vi "Exercise 6.1 RT PID-DataLog - LED.vi"() -> ()   [LabVIEW 2014]
doc: "This example demonstrates how to simulate a general PID controller with alarms."
uses:
  <vilib>/platform/TimedLoop/XDataNode/XDataNode.xnode
  <vilib>/Platform/TimedLoop/XDataNode/nitl_modes.ctl
  <vilib>/Platform/TimedLoop/XDataNode/XDNodeRunTimeDep.lvlib
  <vilib>/Platform/TimedLoop/XDataNode/wakeup.ctl
  <vilib>/Platform/TimedLoop/XDataNode/timing_clust.ctl
  <vilib>/Utility/file.llb/Write To Spreadsheet File (DBL).vi
  <vilib>/NI/Current Value Table/Current Value Table.lvlib
  <vilib>/NI/Current Value Table/Type Defs/File Format.ctl
  <vilib>/NI/Current Value Table/DataTypes/Double_Read.vi
  <vilib>/NI/Current Value Table/DataTypes/Double_Write.vi
  <vilib>/NI/Current Value Table/DataTypes/Boolean_Write.vi
  <vilib>/NI/Current Value Table/DataTypes/Boolean_Read.vi
  <vilib>/NI/STM/NI STM.lvlib
  <vilib>/NI/STM/TCP/Write Message (TCP).vi
  <vilib>/Q-Wave Systems/QwaveSys RPi Training Package (Demo)/Exercises/Exercise 6 Network Communucation/LogData.vi
  <vilib>/Utility/file.llb/Write To Spreadsheet File (string).vi
  <vilib>/Q-Wave Systems/QwaveSys RPi Training Package (Demo)/Addons/QwaveSys RPi Training Library.lvlib
  <vilib>/NI/STM/TCP/Write Meta Data (TCP Ref).vi
  <vilib>/NI/STM/TCP/Get Connection Reference (TCP).vi
  <vilib>/NI/Current Value Table/Type Defs/Tag Grouping set.ctl
  <vilib>/NI/Current Value Table/Type Defs/Data Types.ctl
  <vilib>/NI/Current Value Table/Type Defs/Single Tag.ctl
  <vilib>/Q-Wave Systems/QwaveSys RPi Training Package (Demo)/Addons/WiringPi/WiringPi Pin Mode.ctl
  <vilib>/Q-Wave Systems/QwaveSys RPi Training Package (Demo)/Addons/WiringPi/WiringPi GPIO TypeDef.ctl
panel:
  in  "Data Log Rate (ms)":u32=5000
  out "DataLog Loop stop":bool
  out "Network Loop stop":bool
  out "PID Loop stop":bool
  out "Data Log Loop ms":u32=5001
  out "Network Loop ms":u32=100
  out "PID Loop ms":u32=20
  in  "stop":bool
  in  "LED2":T1=5 items=["Pin1_3.3V"=51, "Pin2_5V"=52, "Pin3_GPIO8_I2C1_SDA"=8, "Pin4_5V"=53, "Pin5_GPIO9_I2C1_SCL"=9, "Pin6_Gnd"=54, "Pin7_GPIO7_GPCLK0"=7, "Pin8_GPIO15_TXD_UART"=15, "Pin9_Gnd"=55, "Pin10_GPIO16_RXD_UART"=16, "Pin11_GPIO0"=0, "Pin12_GPIO1_PCMCLK_PWM0"=1, "Pin13_GPIO2"=2, "Pin14_Gnd"=56, "Pin15_GPIO3"=3, "Pin16_GPIO4"=4, "Pin17_3V"=57, "Pin18_GPIO5"=5, "Pin19_GPIO12_MOSI(SPI)"=12, "Pin20_Gnd"=58, "Pin21_GPIO13_MISO(SPI)"=13, "Pin22_GPIO6"=6, "Pin23_GPIO14_CLK(SPI)"=14, "Pin24_GPIO10_CE0_SPI"=10, "Pin25_Gnd"=59, "Pin26_GPIO11_CE1_SPI"=11, "Pin27_SDA0_I2C_EEPROM"=60, "Pin28_SCL0_I2C_EEPROM"=61, "Pin_29_GPIO21_GPCLK1"=21, "Pin30_Gnd"=62, "Pin31_GPIO22_GPCLK2"=22, "Pin32_GPIO26_PWM0"=26, "Pin33_GPIO23_PWM1"=23, "Pin34_Gnd"=63, "Pin35_GPIO24_PCMFS_PWM1"=24, "Pin36_GPIO27"=27, "Pin37_GPIO25"=25, "Pin38_GPIO28_PCM_DIN"=28, "Pin39_Gnd"=64, "Pin40_GPIO29_PCM_DOUT"=29]
  in  "LED1":T1=1 items=["Pin1_3.3V"=51, "Pin2_5V"=52, "Pin3_GPIO8_I2C1_SDA"=8, "Pin4_5V"=53, "Pin5_GPIO9_I2C1_SCL"=9, "Pin6_Gnd"=54, "Pin7_GPIO7_GPCLK0"=7, "Pin8_GPIO15_TXD_UART"=15, "Pin9_Gnd"=55, "Pin10_GPIO16_RXD_UART"=16, "Pin11_GPIO0"=0, "Pin12_GPIO1_PCMCLK_PWM0"=1, "Pin13_GPIO2"=2, "Pin14_Gnd"=56, "Pin15_GPIO3"=3, "Pin16_GPIO4"=4, "Pin17_3V"=57, "Pin18_GPIO5"=5, "Pin19_GPIO12_MOSI(SPI)"=12, "Pin20_Gnd"=58, "Pin21_GPIO13_MISO(SPI)"=13, "Pin22_GPIO6"=6, "Pin23_GPIO14_CLK(SPI)"=14, "Pin24_GPIO10_CE0_SPI"=10, "Pin25_Gnd"=59, "Pin26_GPIO11_CE1_SPI"=11, "Pin27_SDA0_I2C_EEPROM"=60, "Pin28_SCL0_I2C_EEPROM"=61, "Pin_29_GPIO21_GPCLK1"=21, "Pin30_Gnd"=62, "Pin31_GPIO22_GPCLK2"=22, "Pin32_GPIO26_PWM0"=26, "Pin33_GPIO23_PWM1"=23, "Pin34_Gnd"=63, "Pin35_GPIO24_PCMFS_PWM1"=24, "Pin36_GPIO27"=27, "Pin37_GPIO25"=25, "Pin38_GPIO28_PCM_DIN"=28, "Pin39_Gnd"=64, "Pin40_GPIO29_PCM_DOUT"=29]
  in  "Pin Mode":T2=enum."OUTPUT"
  in  "MIN":dbl(slide)=25.510204081632654 scale=0.0..100.0
  in  "MAX":dbl(slide)=74.48979591836735 scale=0.0..100.0
  out "Low Limit":bool
  out "High Limit":bool
  in  "SP:":dbl(slide)=54.966887417218544 min=0.0 max=0.0 scale=0.0..100.0
  out "MV:":dbl(slide)=100.0 scale=-100.0..100.0
  out "PV:":dbl(slide)=33.01408837398299 scale=0.0..100.0
  in  "PID gains":T3={"proportional gain (Kc)"=20.0, "integral time (Ti, min)"=0.008, "derivative time (Td, min)"=0.001} {"derivative time (Td, min)" format="%.3f"; "integral time (Ti, min)" format="%.3f"; "proportional gain (Kc)" format="%.3f"}
  # "Overview: This example demonstrates how to simulate a general PID controller with alarms.\nInstructions:\n1. Run the VI and observe the Process Variable (PV) following the Setpoint (SP) value.\n2. Move the setpoint above or below the High Limit (HL) or Low Limit (LL). Verify the controls flashing when limits are reached.\n3. Change the Alarm limits to a value above or below if you are changing HL or LL, respectively and verify that the controller stop flashing.\n3. Click Stop to stop the VI."
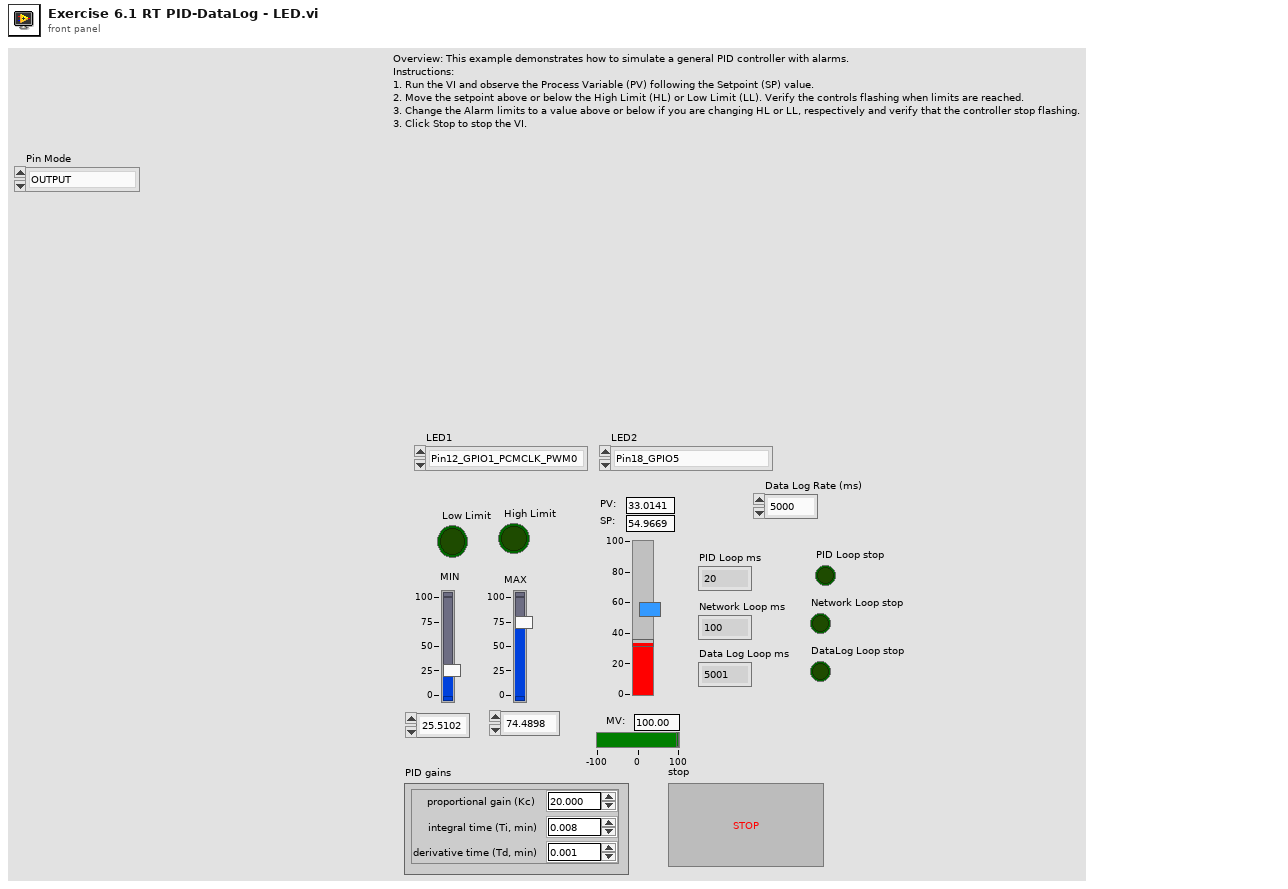
[diagram p1: front panel]
types:
  T1 = typedef "QwaveSys RPi Training Library.lvlib/WiringPi GPIO TypeDef.ctl" = u8
  T2 = typedef "QwaveSys RPi Training Library.lvlib/WiringPi Pin Mode.ctl" = enum8{"INPUT", "OUTPUT", "PWM_OUTPUT", "GPIO_CLOCK", "SOFT_PWM_OUTPUT", "SOFT_TONE_OUTPUT", "PWM_TONE_OUTPUT"}
  T3 = cluster{"proportional gain (Kc)":dbl, "integral time (Ti, min)":dbl, "derivative time (Td, min)":dbl}
  T4 = typedef "Current Value Table.lvlib/File Format.ctl" = cluster{"Tags":T5[], "Group Listings":T7[]}
  T5 = typedef "Current Value Table.lvlib/Single Tag.ctl" = cluster{"Data Type":T6, "Name":string, "Value":string, "Description":string}
  T6 = typedef "Current Value Table.lvlib/Data Types.ctl" = enum16{"Double", "Single", "I64", "I32", "I16", "I8", "U64", "U32", "U16", "U8", "String", "Boolean", "Array of U8", "Array of U16", "Array of U32", "Array of U64", "Array of I64", "Array of I32", "Array of I16", "Array of I8", "Array of Double", "Array of Single", "Array of Boolean", "Array of String"}
  T7 = typedef "Current Value Table.lvlib/Tag Grouping set.ctl" = cluster{"Group":string, "Tag Names":string[]}
  T8 = typedef "NI STM.lvlib/TCP Connection Info.ctl" = cluster{"connection ID":refnum<k5>, "meta data":T9[]}
  T9 = typedef "NI STM.lvlib/MetaDataElement.ctl" = string
  T10 = typedef "XDNodeRunTimeDep.lvlib/timing_clust.ctl" = cluster{"Expected End [f-1]":u64, "Actual End [f-1]":u64, "Finished Late? [f-1]":bool, "Expected End [i-1]":u64, "Actual End [i-1]":u64, "Finished Late? [i-1]":bool, "Expected Start [i]":u64, "Actual Start [i]":u64, "Expected Start [f]":u64, "Actual Start [f]":u64, "Source Name":string, "Structure Name":string, "Period":i64, "Deadline":i64, "Offset":i64, "Start":i64, "Priority":i32, "Timeout":i32, "Mode":T11, "Wakeup Reason":T12, "Error":errorcluster, "Source Type":string, "Secondary Source Type":string, "Global End Time":u64, "Global Start Time":u64, "Frame Duration":u64, "Iteration Duration":u64, "Assigned CPU":i32, "I/O Scan Engine Mode":u32}
  T11 = typedef "XDNodeRunTimeDep.lvlib/nitl_modes.ctl" = enum32{"No Change", "Process missed periods, maintain original phase", "Discard missed periods, maintain original phase", "Process missed periods, ignore original phase", "Discard missed periods, ignore original phase"}
  T12 = typedef "XDNodeRunTimeDep.lvlib/wakeup.ctl" = enum32{"Normal", "Aborted", "Asynchronous wakeup", "Timing source error", "Timed loop error", "Timeout"}
  T13 = cluster{"static gain":dbl, "lag (min)":dbl, "dead cycles":dbl, "load %":dbl, "deadband":dbl, "noise level %":dbl, "initial PV":dbl, "initial PV 2":dbl}
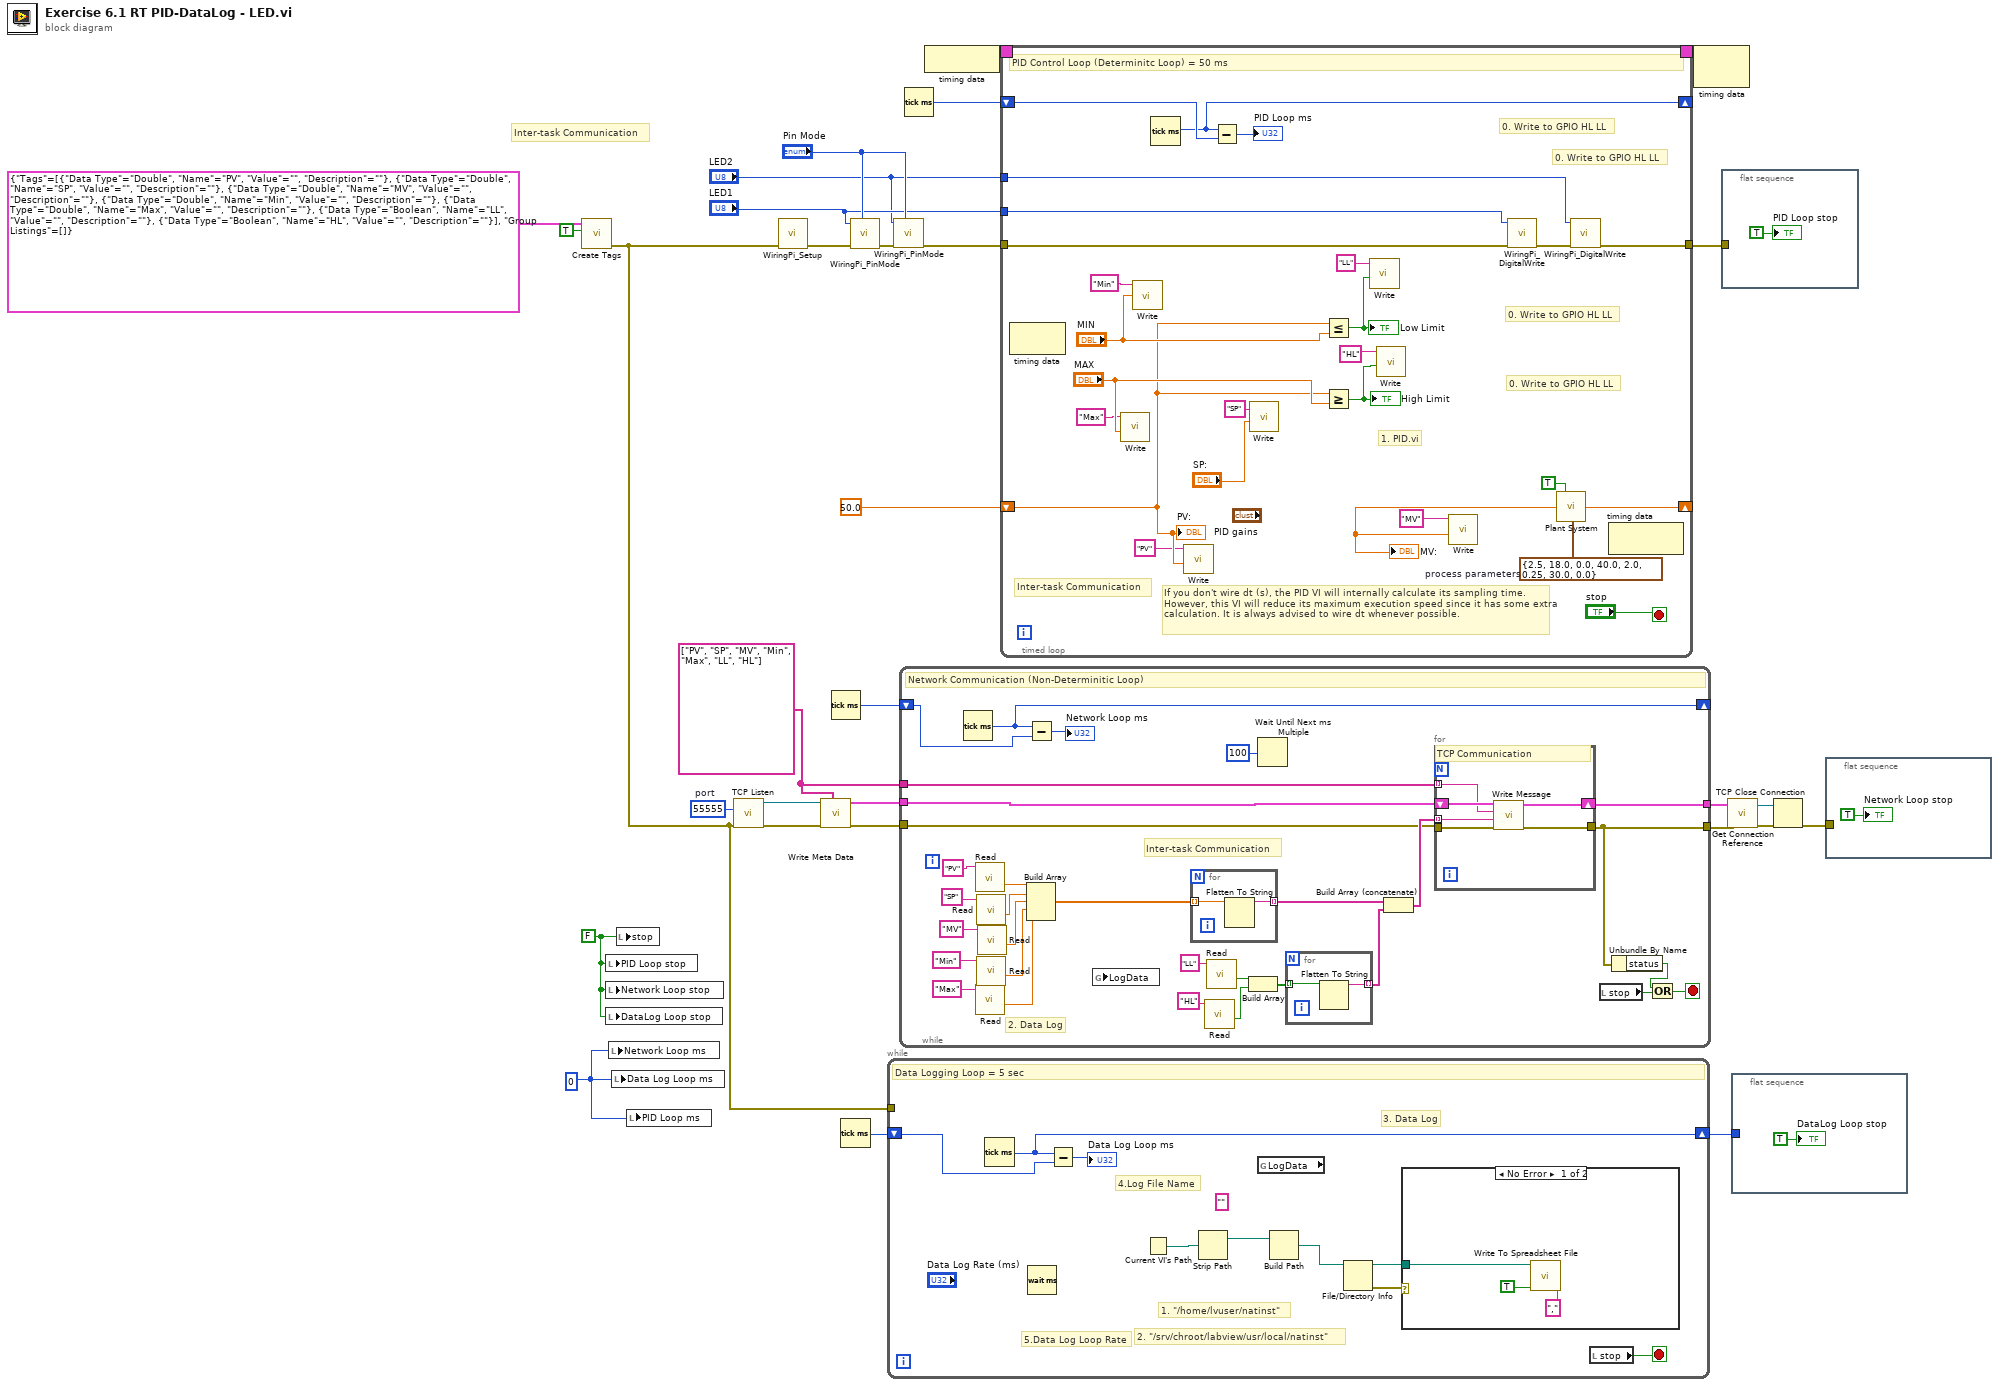
[diagram p0: block diagram]
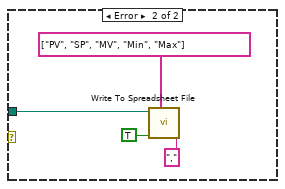
[diagram p2: hidden frame]
diagram:
  w2 = 0
  w3 = FALSE ("stop")
  w20 = string[] ["PV", "SP", "MV", "Min", "Max", "LL", "HL"] ("Meta data")
  w27 = u16 55555  # port
  # "Inter-task Communication"
  n1 = call <vilib>:"Create Tags.vi"("Clear Table? (F)"=TRUE, "CVT Tags to Create"=T4 {"Tags"=[{"Data Type"=enum."Double", "Name"="PV", "Value"="", "Description"=""}, {"Data Type"=enum."Double", "Name"="SP", "Value"="", "Description"=""}, {"Data Type"=enum."Double", "Name"="MV", "Value"="", "Description"=""}, {"Data Type"=enum."Double", "Name"="Min", "Value"="", "Description"=""}, {"Data Type"=enum."Double", "Name"="Max", "Value"="", "Description"=""}, {"Data Type"=enum."Boolean", "Name"="LL", "Value"="", "Description"=""}, {"Data Type"=enum."Boolean", "Name"="HL", "Value"="", "Description"=""}], "Group Listings"=[]}) -> ("error out"=w1:errorcluster)  [unwired: 9 in]
  n2 = local write "PID Loop stop"(w3) -> ()
  n3 = local write "Network Loop stop"(w3) -> ()
  n4 = local write "DataLog Loop stop"(w3) -> ()
  n5 = local write "Network Loop ms"(w2) -> ()
  n6 = local write "Data Log Loop ms"(w2) -> ()
  n7 = local write "stop"(w3) -> ()
  n8 = local write "PID Loop ms"(w2) -> ()
  n9 = call <vilib>:"TCP Listen.vi"("error in (no error)"=w1, "port"=w27) -> ("error out"=w10:errorcluster, "connection ID"=w26:refnum<k5>)  [unwired: 2 in, 6 out]
  n10 = call <vilib>:"WiringPi_Setup.vi"("error in (no error)"=w1) -> ("error out"=w16:errorcluster)  [unwired: 10 in]
  n11 = call-poly <vilib>:"Write Meta Data.vi"("meta data"=w20, "error in"=w10, "connection ID"=w26) -> ("error out"=w17:errorcluster, "connection info out"=w25:T8)  [unwired: 7 in]
  n12 = Tick Count (ms)() -> (millisecond timer value=w8:u32)
  n13 = Tick Count (ms)() -> (millisecond timer value=w7:u32)
  n14 = call <vilib>:"WiringPi_PinMode.vi"("Pin Mode"="Pin Mode", "error in (no error)"=w16, "WiringPi GPIO"="LED1") -> ("error out"=w14:errorcluster)  [unwired: 8 in]
  n15 = while {
    tunnel: w1 -> [_]
    shift-right: [w31] -> w4
    shift-left: w7 -> [w32]
    stop <- w34 stop-if-true
    (unwired) "" ("Log File Name .xxx")
    # "5.Data Log Loop Rate"
    # "4.Log File Name"
    # "3. Data Log"
    # "1. \"/home/lvuser/natinst\""
    # "2. \"/srv/chroot/labview/usr/local/natinst\""
    # "Data Logging Loop = 5 sec"
    n16 = Tick Count (ms)() -> (millisecond timer value=w31:u32)
    n17 = Wait (ms)() -> ()  [unwired: 1 in, 1 out]
    n18 = Subtract(x=w31, y=w32) -> (x-y=→"Data Log Loop ms":u32)
    n19 = Current VI's Path() -> (path=w39:path)
    n20 = Strip Path(path=w39) -> (stripped path=w38:path)  [unwired: 1 out]
    n21 = global read "LogData.vi" "LogData"() -> ()  [unwired: 1 out]
    n22 = Build Path(base path=w38) -> (appended path=w37:path)  [unwired: 1 in]
    n23 = File/Directory Info(path=w37) -> (path out=w35:path, error out=w36:errorcluster)  [unwired: 1 in, 5 out]
    n24 = case shown="No Error" w36 {
      tunnel: w35 -> [w40 w44]
      frame No Error {
        n25 = call-poly <vilib>:"Write To Spreadsheet File.vi"("delimiter (\\t)"="," ("delimiter (\\t)"), "append to file? (new file:F)"=TRUE, "file path (dialog if empty)"=w40) -> ()  [unwired: 5 in, 1 out]
      }
      frame Error {
        n26 = call-poly <vilib>:"Write To Spreadsheet File.vi"("delimiter (\\t)"="," ("delimiter (\\t)"), "append to file? (new file:F)"=TRUE, "1D data"=string[] ["PV", "SP", "MV", "Min", "Max"], "file path (dialog if empty)"=w44) -> ()  [unwired: 4 in, 1 out]
      }
    }
    n27 = local read "stop"() -> (w34:bool)
  }
  n28 = call <vilib>:"WiringPi_PinMode.vi"("Pin Mode"="Pin Mode", "error in (no error)"=w14, "WiringPi GPIO"="LED2") -> ("error out"=w13:errorcluster)  [unwired: 8 in]
  n29 = while {
    tunnel: w25 -> [w73]
    tunnel: w17 -> [w68]
    tunnel: [w72] -> w22
    tunnel: [w69] -> w21
    tunnel: w20 -> [w71]
    shift-right: [w48] -> _
    shift-left: w8 -> [w49]
    stop <- w62 stop-if-true
    # "2. Data Log"
    # "Inter-task Communication"
    # "Network Communication (Non-Determinitic Loop)"
    n30 = Tick Count (ms)() -> (millisecond timer value=w48:u32)
    n31 = call-poly <vilib>:"Read.vi"("Tag Name"="PV") -> ("Value"=w56:dbl)  [unwired: 9 in, 1 out]
    n32 = call-poly <vilib>:"Read.vi"("Tag Name"="Max") -> ("Value"=w60:dbl)  [unwired: 9 in, 1 out]
    n33 = call-poly <vilib>:"Read.vi"("Tag Name"="SP") -> ("Value"=w57:dbl)  [unwired: 9 in, 1 out]
    n34 = call-poly <vilib>:"Read.vi"("Tag Name"="Min") -> ("Value"=w59:dbl)  [unwired: 9 in, 1 out]
    n35 = call-poly <vilib>:"Read.vi"("Tag Name"="MV") -> ("Value"=w58:dbl)  [unwired: 9 in, 1 out]
    n36 = Subtract(x=w48, y=w49) -> (x-y=→"Network Loop ms":u32)
    n37 = Build Array(w56, w57, w58, w59, w60) -> (w50:dbl[])
    n38 = global read "LogData.vi" "LogData"() -> ()  [unwired: 1 in]
    n39 = for {
      tunnel: w50 -> [w81] mode=indexing
      tunnel: [w80] -> w77 mode=indexing
      n40 = Flatten To String(anything=w81) -> (data string=w80:string)  [unwired: 1 in, 4 out]
    }
    n41 = call-poly <vilib>:"Read.vi"("Tag Name"="HL") -> ("Value"=w64:bool)  [unwired: 9 in, 1 out]
    n42 = call-poly <vilib>:"Read.vi"("Tag Name"="LL") -> ("Value"=w67:bool)  [unwired: 9 in, 1 out]
    n43 = Build Array(w67, w64) -> (w76:bool[])
    n44 = Wait Until Next ms Multiple(millisecond multiple=u32 100) -> ()  [unwired: 1 out]
    n45 = for {
      tunnel: w76 -> [w79] mode=indexing
      tunnel: [w78] -> w75 mode=indexing
      n46 = Flatten To String(anything=w79) -> (data string=w78:string)  [unwired: 1 in, 4 out]
    }
    n47 = Build Array (concatenate)(w77, w75) -> (w74:string[])
    n48 = for {
      tunnel: [w86] -> w69
      tunnel: w68 -> [w85]
      tunnel: w74 -> [w83] mode=indexing
      shift-right: [w87] -> w72
      shift-left: w73 -> [w84]
      tunnel: w71 -> [w82] mode=indexing
      # "TCP Communication"
      n49 = call-poly <vilib>:"Write Message.vi"("error in"=w85, "data"=w83, "name"=w82, "connection info in"=w84) -> ("error out"=w86:errorcluster, "connection info out"=w87:T8)  [unwired: 6 in]
    }
    n50 = local read "stop"() -> (w63:bool)
    n51 = Unbundle By Name(w69) -> ("status"=w61:bool)
    n52 = Or(x=w61, y=w63) -> (x .or. y?=w62:bool)
  }
  n53 = Tick Count (ms)() -> (millisecond timer value=w9:u32)
  n54 = node-c288() -> (w29:T10)
  n55 = timed-loop {
    shift-left: 50.0 ("Plant Output") -> [w104]
    shift-right: [w113] -> _
    timing: w29 -> [_]
    timing-out: [_] -> w28
    tunnel: w13 -> [w98]
    tunnel: [w96] -> w6
    tunnel: "LED1" -> [w95]
    tunnel: "LED2" -> [w94]
    shift-right: [w89] -> _
    shift-left: w9 -> [w90]
    stop <- "stop" stop-if-true
    w112 = T13 {"static gain"=2.5, "lag (min)"=18.0, "dead cycles"=0.0, "load %"=40.0, "deadband"=2.0, "noise level %"=0.25, "initial PV"=30.0, "initial PV 2"=0.0}  # process parameters
    # "0. Write to GPIO HL LL"
    # "0. Write to GPIO HL LL"
    # "0. Write to GPIO HL LL"
    # "0. Write to GPIO HL LL"
    # "1. PID.vi"
    # "Inter-task Communication"
    # "If you don't wire dt (s), the PID VI will internally calculate its sampling time. However, this VI will reduce its maximum execution speed since it has some extra calculation. It is always advised to wire dt whenever possible."
    # "PID Control Loop (Determinitc Loop) = 50 ms"
    n56 = node-c288() -> ()  [unwired: 1 in, 1 out]
    n57 = call-poly <vilib>:"Write.vi"("Value"="MAX", "Tag Name"="Max") -> ()  [unwired: 9 in, 1 out]
    n58 = call-poly <vilib>:"Write.vi"("Value"="MIN", "Tag Name"="Min") -> ()  [unwired: 9 in, 1 out]
    n59 = Tick Count (ms)() -> (millisecond timer value=w89:u32)
    n60 = call-poly <vilib>:"Write.vi"("Value"=w104, "Tag Name"="PV") -> ()  [unwired: 9 in, 1 out]
    n61 = Subtract(x=w89, y=w90) -> (x-y=→"PID Loop ms":u32)
    n62 = call-poly <vilib>:"Write.vi"("Value"="SP:", "Tag Name"="SP") -> ()  [unwired: 9 in, 1 out]
    n63 = Less Or Equal?(x=w104, y="MIN") -> (x <= y?=w93:bool)
    "Low Limit" <- w93
    n64 = Greater Or Equal?(x=w104, y="MAX") -> (x >= y?=w92:bool)
    "High Limit" <- w92
    n65 = call-poly <vilib>:"Write.vi"("Value"=w93, "Tag Name"="LL") -> ()  [unwired: 9 in, 1 out]
    n66 = call-poly <vilib>:"Write.vi"("Value"=w92, "Tag Name"="HL") -> ()  [unwired: 9 in, 1 out]
    n67 = call <vilib>:"WiringPi_DigitalWrite.vi"("error in (no error)"=w98, "WiringPi GPIO"=w95) -> ("error out"=w97:errorcluster)  [unwired: 9 in]
    n68 = call <vilib>:"Plant System.vi"("Integrator ?"=TRUE, "process parameters"=w112) -> ("Plant Input"=w102:dbl, "Plant Output"=w113:dbl)  [unwired: 12 in]
    "MV:" <- w102
    n69 = call-poly <vilib>:"Write.vi"("Value"=w102, "Tag Name"="MV") -> ()  [unwired: 9 in, 1 out]
    n70 = call <vilib>:"WiringPi_DigitalWrite.vi"("error in (no error)"=w97, "WiringPi GPIO"=w94) -> ("error out"=w96:errorcluster)  [unwired: 9 in]
    n71 = node-c288() -> ()  [unwired: 1 in, 1 out]
    "PV:" <- w104
  }
  n72 = node-c288(w28) -> ()  [unwired: 1 out]
  n73 = flat-sequence {
    tunnel: w6 -> [_]
    frame #0 {
      "PID Loop stop" <- TRUE ("PID Loop stop")
    }
  }
  n74 = call-poly <vilib>:"Get Connection Reference.vi"("error in"=w21, "connection info in"=w22) -> ("error out"=w23:errorcluster, "connection ID out"=w24:refnum<k5>)  [unwired: 7 in, 1 out]
  n75 = flat-sequence {
    tunnel: w4 -> [_]
    frame #0 {
      "DataLog Loop stop" <- TRUE ("DataLog Loop stop")
    }
  }
  n76 = TCP Close Connection(connection ID=w24, error in (no error)=w23) -> (error out=w5:errorcluster)  [unwired: 2 out]
  n77 = flat-sequence {
    tunnel: w5 -> [_]
    frame #0 {
      "Network Loop stop" <- TRUE ("Network Loop stop 2")
    }
  }
